vi "Test_PublicationLocked_PublisherOwnsLock_OK.vi"(8 "error in (no error)":errorcluster, 11 "TestMediator In":refnum<class "TestMediationSemantics.lvclass">) -> (0 "error out":errorcluster, 3 "TestMediator Out":refnum<class "TestMediationSemantics.lvclass">)   [LabVIEW 2020, in "TestMediationSemantics.lvclass"]
uses:
  TestMediationSemantics.lvclass
  TestMediationSemantics.lvclass/TestMediationSemantics.ctl
  Source/Mediator/Mediator/Mediator.lvclass
  <vilib>/ActorFramework/Actor/Actor.lvclass
  Source/IMediator/IMediator Messages/Publish Msg/Publish Msg.lvclass
  Source/IMediator/IMediator Messages/Subscribe Msg/Subscribe Msg.lvclass
  Source/IMediator/SubscriptionRequest/SubscriptionRequest.lvclass
  Source/IMediator/ISubscriptionPolicy/ISubscriptionPolicy.lvclass
  <vilib>/ActorFramework/Stop Msg/Stop Msg.lvclass
  Source/SubscriptionPolicy/BasicSubscription/BasicSubscription.lvclass
  Source/IMediator/IMediator Messages/Lock Publication Msg/Lock Publication Msg.lvclass
  modules/composed-transport/Source/Concrete/QueueTransport/QueueTransport.lvclass
  Source/IMediator/PublishRequest/PublishRequest.lvclass
  C:/Git/mva-core/Source/IMediator/IMediator/IMediator.lvclass
  C:/Program Files (x86)/National Instruments/LabVIEW 2020/vi.lib/ActorFramework/Actor/Actor.lvclass
  C:/Git/mva-core/Source/Mediator/Mediator/Mediator.lvclass
  C:/Git/mva-core/Source/IMediator/ISubscriptionPolicy/ISubscriptionPolicy.lvclass
  C:/Git/mva-core/Source/SubscriptionPolicy/BasicSubscription/BasicSubscription.lvclass
  C:/Git/mva-core/modules/composed-transport/Source/ITransport/ITransport.lvclass
  C:/Git/mva-core/modules/composed-transport/Source/Concrete/QueueTransport/QueueTransport.lvclass
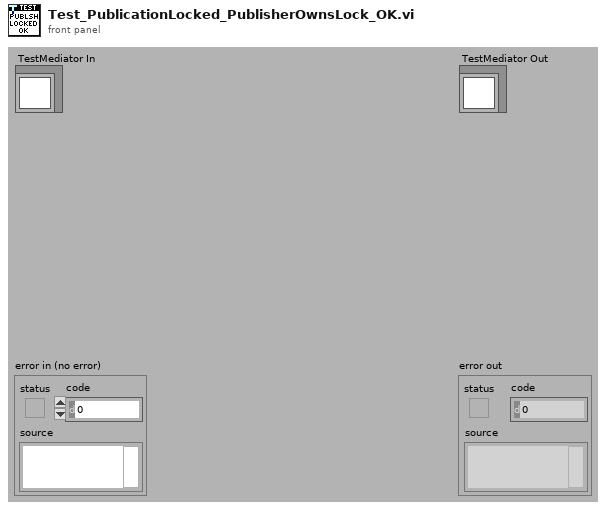
[diagram p1: front panel]
types:
  T1 = typedef "IMediator.lvlib/ISubscriptionPolicy.lvclass/ISubscriptionPolicy Reference.ctl" = refnum<data-value>
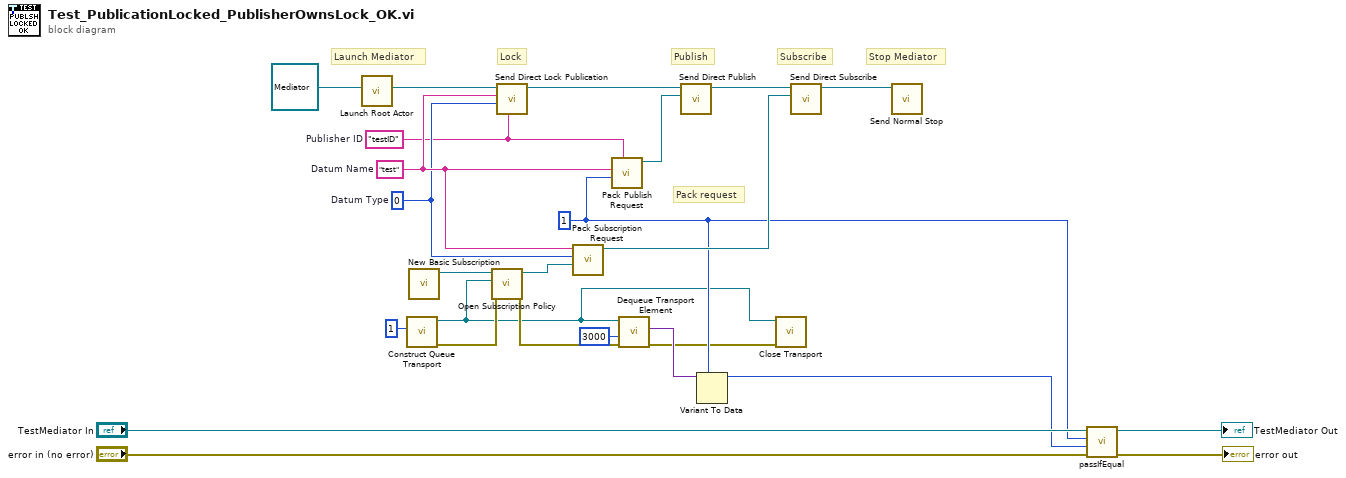
[diagram p0: block diagram]
diagram:
  w3 = "testID"  # Publisher ID
  w4 = 0  # Datum Type
  w5 = "test"  # Datum Name
  w8 = 1
  # "Pack request"
  # "Lock"
  # "Launch Mediator"
  # "Stop Mediator"
  # "Subscribe"
  # "Publish"
  n1 = call <vilib>:"Launch Root Actor.vi"("Actor"=refnum<class "Mediator.lvclass"> refnum ("Mediator.lvlib:Mediator.lvclass")) -> ("Actor's Enqueuer"=w20:refnum<class "Message Enqueuer.lvclass">)  [unwired: 9 in, 1 out]
  n2 = call "Construct Queue Transport.vi"("Max Queue Size (-1)"=1) -> ("error out"=w15:errorcluster, "QueueTransport"=w1:refnum<class "QueueTransport.lvclass">)  [unwired: 9 in]
  n3 = call "New Basic Subscription.vi"() -> ("BasicSubscription Out"=w10:refnum<class "BasicSubscription.lvclass">)  [unwired: 11 in]
  n4 = call "Open Subscription Policy.vi"("error in (no error)"=w15, "Transport"=w1, "SubscriptionPolicy"=w10) -> ("error out"=w14:errorcluster, "Subscription Policy"=w9:T1)  [unwired: 7 in]
  n5 = call "Send Direct Lock Publication.vi"("Publisher ID"=w3, "Datum Type"=w4, "Datum Name"=w5, "Mediator Enqeuer"=w20) -> ("Mediator Enqueuer out"=w6:refnum<class "Message Enqueuer.lvclass">)  [unwired: 6 in, 1 out]
  n6 = call "Pack Subscription Request.vi"("Subscription Policy"=w9, "Type"=w4, "Datum Name"=w5) -> ("SubscriptionRequest"=w19:refnum<class "SubscriptionRequest.lvclass">)  [unwired: 7 in, 1 out]
  n7 = call "Pack Publish Request.vi"("Publisher ID"=w3, "Value"=w8, "Datum Name"=w5) -> ("PublishRequest Out"=w7:refnum<class "PublishRequest.lvclass">)  [unwired: 7 in, 1 out]
  n8 = call "Dequeue Transport Element.vi"("error in (no error)"=w14, "Timeout In ms (-1)"=3000, "QueueTransport"=w1) -> ("error out"=w2:errorcluster, "Data"=w12:variant)  [unwired: 5 in, 2 out]
  n9 = call "Send Direct Publish.vi"("PublishRequest"=w7, "Mediator Enqueuer"=w6) -> ("Mediator Enqueuer out"=w18:refnum<class "Message Enqueuer.lvclass">)  [unwired: 8 in, 1 out]
  n10 = Variant To Data(type=w8, Variant=w12) -> (data=w11:i32)  [unwired: 1 in, 1 out]
  n11 = call-dynamic "Close Transport.vi"("error in (no error)"=w2, "QueueTransport"=w1) -> ()  [unwired: 9 in, 1 out]
  n12 = call "Send Direct Subscribe.vi"("Subscription Request"=w19, "Message Enqueuer"=w18) -> ("Message Enqueuer out"=w13:refnum<class "Message Enqueuer.lvclass">)  [unwired: 8 in, 1 out]
  n13 = call <vilib>:"Send Normal Stop.vi"("Message Enqueuer"=w13) -> ()  [unwired: 10 in, 1 out]
  n14 = call-dynamic "passIfEqual.vi"("error in (no error)"="error in (no error)", "y"=w11, "x"=w8, "TestCase in"="TestMediator In") -> ("error out"=→"error out":errorcluster, "TestCase out"=→"TestMediator Out":refnum<class "TestMediationSemantics.lvclass">)  [unwired: 6 in]
